vi "Read Pressure DBL.vi"(8 "error in":errorcluster, 10 "Source":string, 11 "IRead Pressure in":refnum<class "IRead Pressure.lvclass">) -> (0 "error out":errorcluster, 1 "Time Stamp":timestamp format="%<%x %.3X>T", 2 "Pressure":dbl, 3 "IRead Pressure out":refnum<class "IRead Pressure.lvclass">)   [LabVIEW 2024, in "IRead Pressure.lvclass"]
uses:
  IRead Pressure.lvclass
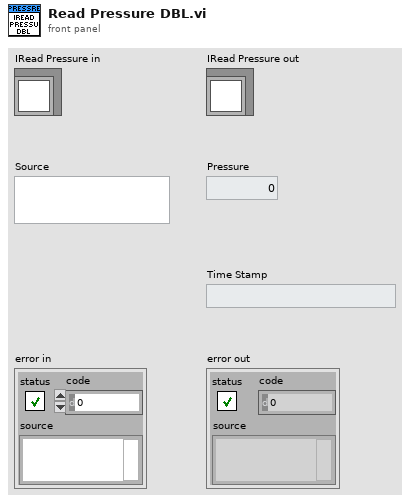
[diagram p1: front panel]
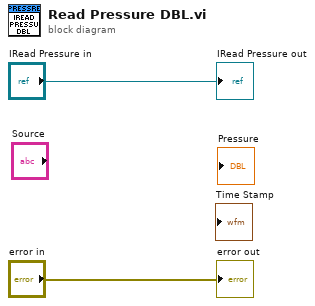
[diagram p0: block diagram]
diagram:
  "error out" <- "error in"
  "IRead Pressure out" <- "IRead Pressure in"
